vi "sv_IMD Product Frequencies.vi"(7 "measurement bandwidth":dbl, 9 "override order":i32=7, 10 "f2":dbl, 11 "f1":dbl) -> (1 "order":i32, 2 "IMD product frequencies":dbl[](array[numeric]), 3 "IMD product frequencies by order":T1(array[cluster]))   [LabVIEW 2017, in "SoundVib_Distortion.lvlib"]
uses:
  <vilib>/addons/Sound and Vibration/svt_Distortion/SoundVib_Distortion.lvlib
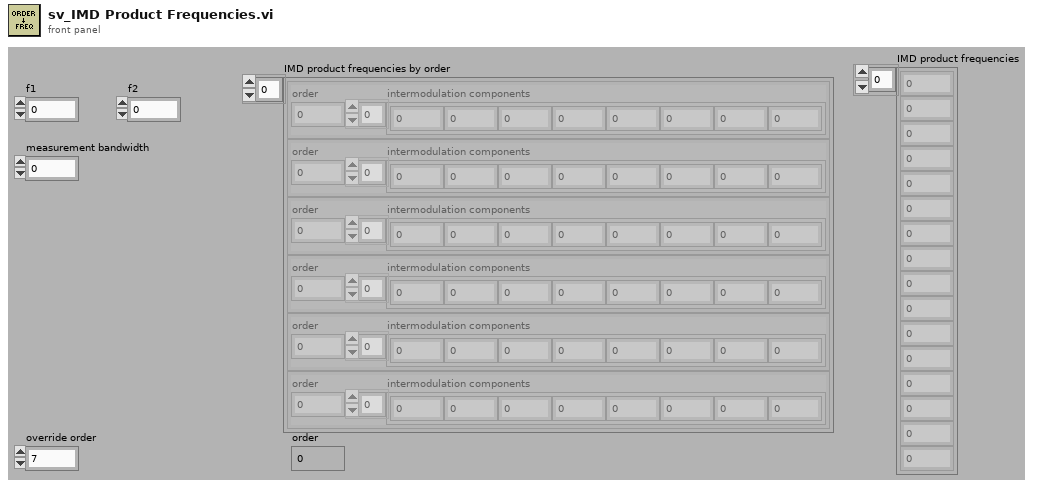
[diagram p1: front panel]
types:
  T1 = cluster{"order":i32, "intermodulation components":dbl[]}[]
  T2 = cluster{"order":i32, "intermodulation components":dbl[]}
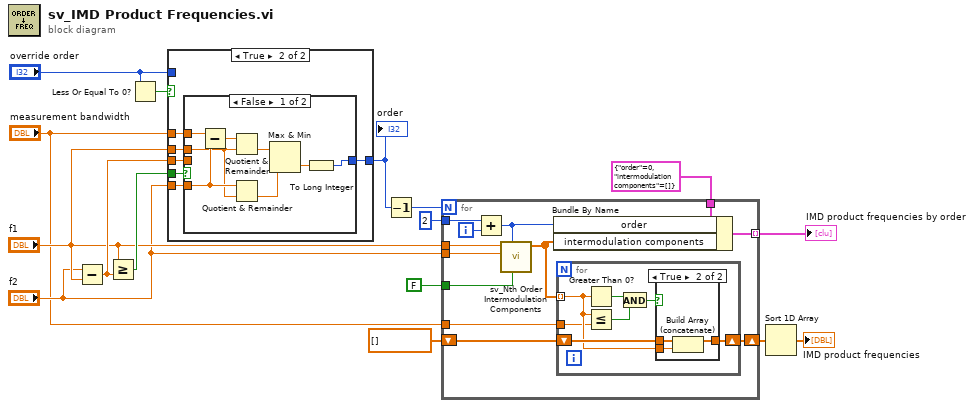
[diagram p0: block diagram]
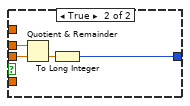
[diagram p3: hidden frame]
diagram:
  n1 = Subtract(x="f2", y="f1") -> (x-y=w15:dbl)
  n2 = Greater Or Equal?(x="f1", y=w15) -> (x >= y?=w16:bool)
  n3 = Less Or Equal To 0?(x="override order") -> (x <= 0?=w13:bool)
  n4 = case shown="True" w13 {
    tunnel: w16 -> [_ w23]
    tunnel: w15 -> [_ w22]
    tunnel: "measurement bandwidth" -> [_ w21]
    tunnel: "f1" -> [_ w20]
    tunnel: "f2" -> [_ w19]
    tunnel: [w17 w18] -> w6
    tunnel: "override order" -> [w17 _]
    frame False {
    }
    frame True {
      n5 = case shown="False" w23 {
        tunnel: w20 -> [w24 w35]
        tunnel: w22 -> [_ w34]
        tunnel: [w25 w32] -> w18
        tunnel: w21 -> [w31 _]
        tunnel: w19 -> [w29 _]
        frame False {
          n6 = Subtract(x=w31, y=w29) -> (x-y=w30:dbl)
          n7 = Quotient & Remainder(x=w30, y=w24) -> (floor(x/y)=w28:dbl)  [unwired: 1 out]
          n8 = Quotient & Remainder(x=w29, y=w24) -> (floor(x/y)=w27:dbl)  [unwired: 1 out]
          n9 = Max & Min(x=w28, y=w27) -> (min(x,y)=w26:dbl)  [unwired: 1 out]
          n10 = To Long Integer(number=w26) -> (32bit integer=w25:i32)
        }
        frame True {
          n11 = Quotient & Remainder(x=w35, y=w34) -> (floor(x/y)=w33:dbl)  [unwired: 1 out]
          n12 = To Long Integer(number=w33) -> (32bit integer=w32:i32)
        }
      }
    }
  }
  "order" <- w6
  n13 = Decrement(x=w6) -> (x-1=w7:i32)
  n14 = for {
    N: w7 -> [_]
    tunnel: "f2" -> [w47]
    tunnel: "f1" -> [w46]
    tunnel: FALSE ("include harmonics") -> [w44]
    tunnel: 2 ("x") -> [w43]
    tunnel: "measurement bandwidth" -> [w42]
    shift-right: [w40] -> w4
    shift-left: dbl[] [] -> [w41]
    tunnel: [w37] -> w2 mode=indexing
    tunnel: T2 {"order"=0, "intermodulation components"=[]} -> [w36]
    i -> [w45]
    n15 = Add(x=w43, y=w45) -> (x+y=w39:i32)
    n16 = call <vilib>:"sv_Nth Order Intermodulation Components.vi"("include harmonics"=w44, "order"=w39, "f2"=w47, "f1"=w46) -> ("Nth order intermodulation components"=w38:dbl[])  [unwired: 7 in]
    n17 = Bundle By Name(cluster=w36, "order"=w39, "intermodulation components"=w38) -> (w37:T2)
    n18 = for {
      tunnel: w38 -> [w52] mode=indexing
      shift-right: [w54] -> w40
      shift-left: w41 -> [w53]
      tunnel: w42 -> [w51]
      n19 = Greater Than 0?(x=w52) -> (x > 0?=w50:bool)
      n20 = Less Or Equal?(x=w52, y=w51) -> (x <= y?=w49:bool)
      n21 = And(x=w50, y=w49) -> (x .and. y?=w48:bool)
      n22 = case shown="True" w48 {
        tunnel: [w55 w56] -> w54
        tunnel: w52 -> [_ w58]
        tunnel: w53 -> [w55 w57]
        frame False {
        }
        frame True {
          n23 = Build Array (concatenate)(w57, w58) -> (w56:dbl[])
        }
      }
    }
  }
  "IMD product frequencies by order" <- w2
  n24 = Sort 1D Array(array=w4) -> (sorted array=→"IMD product frequencies":dbl[])
